vi "2.1.vi"() -> ()   [LabVIEW 2020]
panel:
  out "Array":i32[](array[numeric])
  in  "TAMAÑO":i32
  # "SERIE DE FIBONACCI"
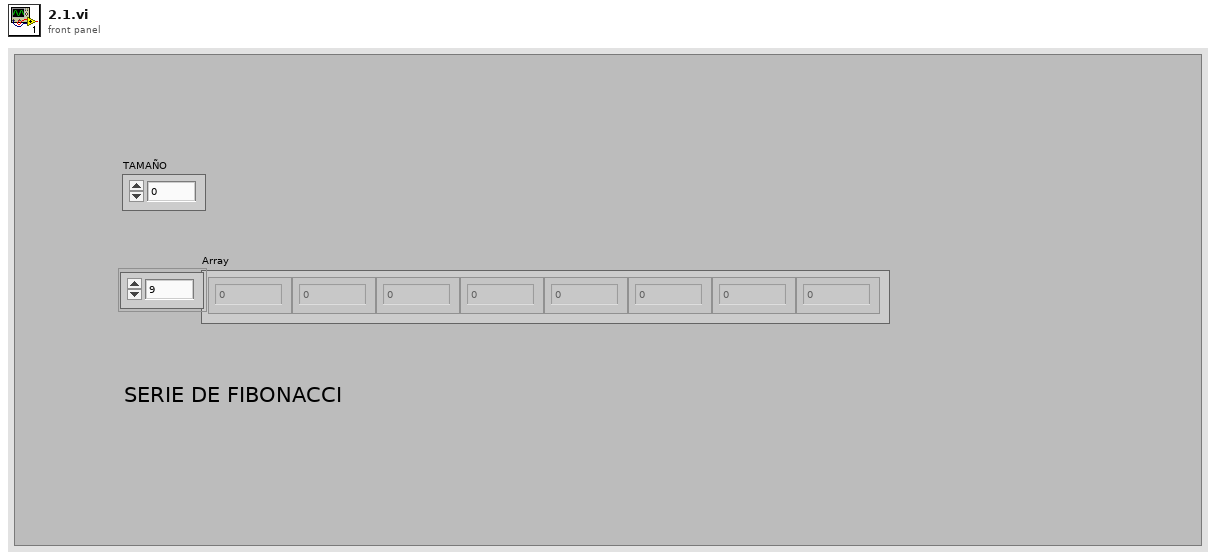
[diagram p1: front panel]
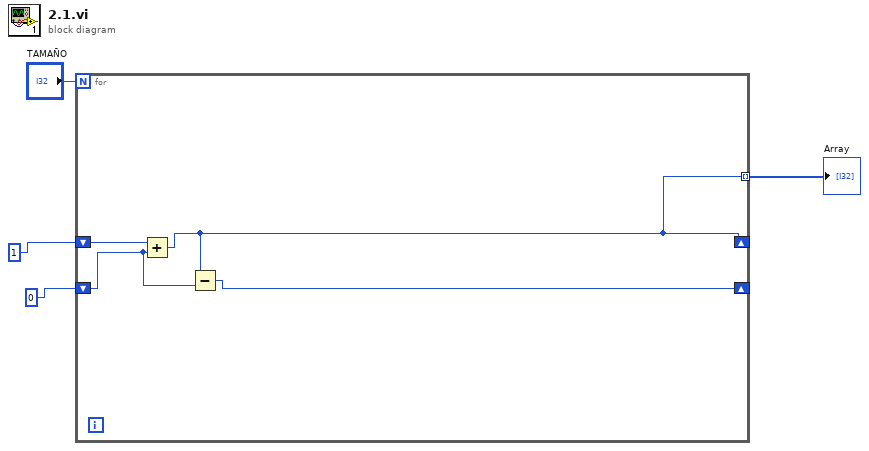
[diagram p0: block diagram]
diagram:
  n1 = for {
    N: "TAMAÑO" -> [_]
    shift-right: [w5] -> _
    shift-left: 1 -> [w8]
    shift-right: [w6] -> _
    shift-left: 0 -> [w7]
    tunnel: [w5] -> w1 mode=indexing
    n2 = Add(x=w8, y=w7) -> (x+y=w5:i32)
    n3 = Subtract(x=w5, y=w7) -> (x-y=w6:i32)
  }
  "Array" <- w1
